vi "Calc_J.vi"(6 "p":dbl[](array[numeric]), 8 "re":dbl, 9 "rf":dbl, 10 "e":dbl, 11 "f":dbl) -> (2 "exist":bool, 3 "theta":dbl)   [LabVIEW 2013]
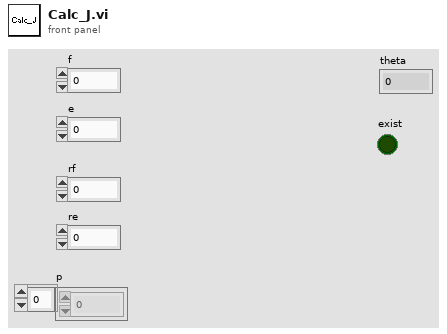
[diagram p1: front panel]
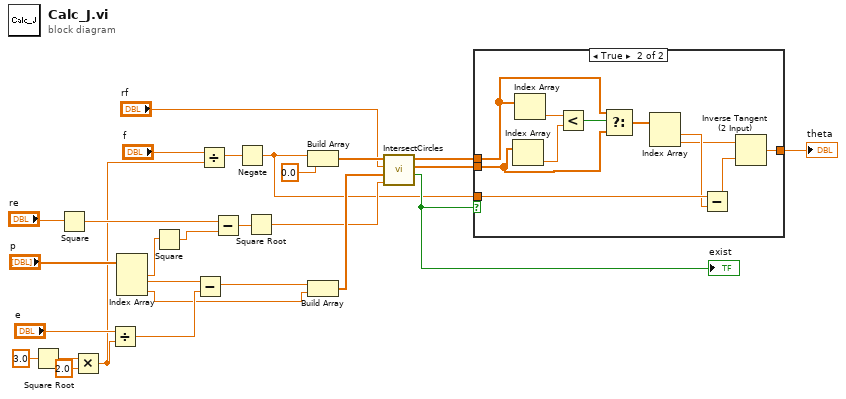
[diagram p0: block diagram]
diagram:
  n1 = Square Root(x=3.0) -> (sqrt(x)=w26:dbl)
  n2 = Square(x="re") -> (x^2=w18:dbl)
  n3 = Multiply(x=w26, y=2.0) -> (x*y=w12:dbl)
  n4 = Divide(x="e", y=w12) -> (x/y=w20:dbl)
  n5 = Index Array(array="p") -> (element #1=w17:dbl, element #2=w22:dbl, element #3=w10:dbl)  [unwired: 3 in]
  n6 = Square(x=w17) -> (x^2=w16:dbl)
  n7 = Subtract(x=w22, y=w20) -> (x-y=w11:dbl)
  n8 = Divide(x="f", y=w12) -> (x/y=w3:dbl)
  n9 = Subtract(x=w18, y=w16) -> (x-y=w15:dbl)
  n10 = Negate(x=w3) -> (-x=w1:dbl)
  n11 = Square Root(x=w15) -> (sqrt(x)=w7:dbl)
  n12 = Build Array(w1, 0.0 ("element")) -> (w13:dbl[])
  n13 = Build Array(w11, w10) -> (w9:dbl[])
  n14 = call "IntersectCircles.vi"("r 1"=w7, "c 1"=w9, "r 0"="rf", "c 0"=w13) -> ("exist"=w4:bool, "p 1"=w5:dbl[], "p 0"=w6:dbl[])  [unwired: 5 in]
  "exist" <- w4
  n15 = case shown="True" w4 {
    tunnel: w6 -> [_ w35]
    tunnel: w5 -> [_ w34]
    tunnel: w1 -> [_ w32]
    tunnel: [_ w28] -> w2
    frame False {
    }
    frame True {
      n16 = Index Array(array=w34) -> (element=w37:dbl)  [unwired: 1 in]
      n17 = Index Array(array=w35) -> (element=w38:dbl)  [unwired: 1 in]
      n18 = Less?(x=w38, y=w37) -> (x < y?=w36:bool)
      n19 = Select(t=w35, s=w36, f=w34) -> (s? t:f=w33:dbl[])
      n20 = Index Array(array=w33) -> (element #1=w31:dbl, element #2=w30:dbl)  [unwired: 2 in]
      n21 = Subtract(x=w32, y=w31) -> (x-y=w29:dbl)
      n22 = Inverse Tangent (2 Input)(1:w29, 2:w30) -> (0:w28:dbl)
    }
  }
  "theta" <- w2
